vi "Color Pulse.vi"(4 "Color 2":u32(colorbox)=16711680, 5 "Style":enum16{"Sine", "Square", "Sawtooth", "Triangle"}(ring), 6 "Color 1":u32(colorbox)=16738922, 7 "Array":refnum<vi>[](array[refnum]), 10 "Pulse Period":dbl, 11 "Elapsed Time (s)":dbl) -> (2 "Color Out":u32(colorbox))   [LabVIEW 2013]
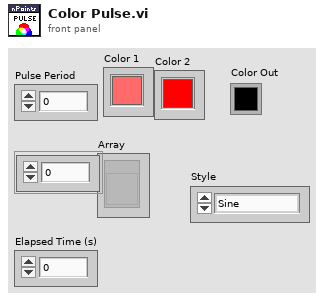
[diagram p1: front panel]
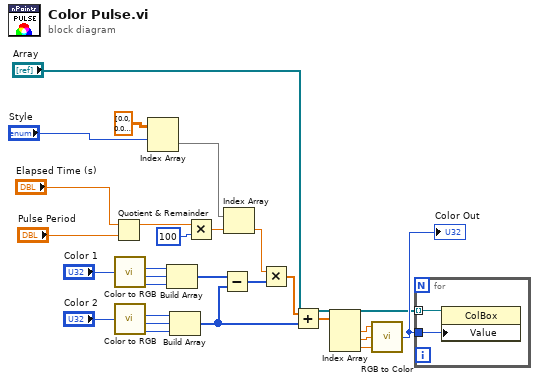
[diagram p0: block diagram]
diagram:
  n1 = Quotient & Remainder(x="Elapsed Time (s)", y="Pulse Period") -> (x-y*floor(x/y)=w23:dbl)  [unwired: 1 out]
  n2 = call <vilib>:"Color to RGB.vi"("Color"="Color 1") -> ("R"=w11:u8, "G"=w12:u8, "B"=w13:u8)  [unwired: 1 out]
  n3 = call <vilib>:"Color to RGB.vi"("Color"="Color 2") -> ("R"=w8:u8, "G"=w9:u8, "B"=w10:u8)  [unwired: 1 out]
  n4 = Index Array(array=dbl[][] [[0.0, 0.0009866357858642205, 0.0039426493427611176, 0.00885637463565564, 0.015708419435684462, 0.02447174185242318, 0.035111757055874326, 0.04758647376699021, 0.061846659978068264, 0.07783603724899246, 0.09549150281252633, 0.11474337861210537, 0.13551568628929428, 0.15772644703565564, 0.18128800512565518, 0.20610737385376343, 0.23208660251050173, 0.2591231629491424, 0.2871103542174637, 0.31593772365766104, 0.34549150281252633, 0.3756550564175726, 0.4063093427071377, 0.43733338321784787, 0.4686047402353434, 0.5, 0.5313952597646567, 0.5626666167821521, 0.5936906572928624, 0.6243449435824274, 0.6545084971874737, 0.684062276342339, 0.7128896457825363, 0.7408768370508576, 0.7679133974894983, 0.7938926261462366, 0.8187119948743449, 0.8422735529643444, 0.8644843137107058, 0.8852566213878946, 0.9045084971874737, 0.9221639627510075, 0.9381533400219317, 0.9524135262330098, 0.9648882429441257, 0.9755282581475768, 0.9842915805643155, 0.9911436253643444, 0.9960573506572389, 0.9990133642141358, 1.0, 0.9990133642141358, 0.9960573506572389, 0.9911436253643444, 0.9842915805643155, 0.9755282581475768, 0.9648882429441257, 0.9524135262330098, 0.9381533400219317, 0.9221639627510076, 0.9045084971874737, 0.8852566213878947, 0.8644843137107058, 0.8422735529643444, 0.8187119948743449, 0.7938926261462367, 0.7679133974894983, 0.7408768370508577, 0.7128896457825363, 0.6840622763423391, 0.6545084971874737, 0.6243449435824274, 0.5936906572928624, 0.5626666167821521, 0.5313952597646567, 0.5000000000000001, 0.4686047402353434, 0.4373333832178479, 0.40630934270713776, 0.3756550564175727, 0.3454915028125264, 0.3159377236576611, 0.2871103542174638, 0.2591231629491424, 0.23208660251050178, 0.2061073738537635, 0.18128800512565524, 0.1577264470356557, 0.13551568628929433, 0.11474337861210543, 0.09549150281252639, 0.07783603724899252, 0.06184665997806832, 0.04758647376699027, 0.03511175705587438, 0.024471741852423234, 0.015708419435684517, 0.008856374635655695, 0.003942649342761173, 0.0009866357858642205], [0.0, 0.0, 0.0, 0.0, 0.0, 0.0, 0.0, 0.0, 0.0, 0.0, 0.0, 0.0, 0.0, 0.0, 0.0, 0.0, 0.0, 0.0, 0.0, 0.0, 0.0, 0.0, 0.0, 0.0, 0.0, 0.0, 0.0, 0.0, 0.0, 0.0, 0.0, 0.0, 0.0, 0.0, 0.0, 0.0, 0.0, 0.0, 0.0, 0.0, 0.0, 0.0, 0.0, 0.0, 0.0, 0.0, 0.0, 0.0, 0.0, 0.0, 1.0, 1.0, 1.0, 1.0, 1.0, 1.0, 1.0, 1.0, 1.0, 1.0, 1.0, 1.0, 1.0, 1.0, 1.0, 1.0, 1.0, 1.0, 1.0, 1.0, 1.0, 1.0, 1.0, 1.0, 1.0, 1.0, 1.0, 1.0, 1.0, 1.0, 1.0, 1.0, 1.0, 1.0, 1.0, 1.0, 1.0, 1.0, 1.0, 1.0, 1.0, 1.0, 1.0, 1.0, 1.0, 1.0, 1.0, 1.0, 1.0, 1.0], [0.0, 0.010000000000000009, 0.019999999999999962, 0.030000000000000027, 0.040000000000000036, 0.050000000000000044, 0.06, 0.07, 0.08000000000000007, 0.09000000000000002, 0.10000000000000003, 0.10999999999999999, 0.12, 0.13000000000000006, 0.14, 0.15000000000000002, 0.16000000000000003, 0.16999999999999998, 0.18000000000000005, 0.19000000000000006, 0.2, 0.21000000000000002, 0.21999999999999997, 0.23000000000000004, 0.24, 0.25, 0.2600000000000001, 0.27, 0.28, 0.29, 0.30000000000000004, 0.31000000000000005, 0.32, 0.33000000000000007, 0.33999999999999997, 0.35000000000000003, 0.3600000000000001, 0.37, 0.38000000000000006, 0.38999999999999996, 0.4, 0.4100000000000001, 0.42, 0.43000000000000005, 0.43999999999999995, 0.45000000000000007, 0.4600000000000001, 0.47000000000000003, 0.4800000000000001, 0.49, 0.5, 0.51, 0.52, 0.53, 0.5399999999999999, 0.55, 0.56, 0.57, 0.5800000000000001, 0.59, 0.6, 0.6100000000000001, 0.62, 0.63, 0.6399999999999999, 0.65, 0.66, 0.6699999999999999, 0.68, 0.69, 0.7, 0.7100000000000001, 0.72, 0.73, 0.74, 0.75, 0.76, 0.77, 0.78, 0.79, 0.8, 0.81, 0.8200000000000001, 0.8300000000000001, 0.8400000000000001, 0.8500000000000001, 0.8600000000000001, 0.87, 0.8800000000000001, 0.8900000000000001, 0.9, 0.9100000000000001, 0.9199999999999999, 0.9299999999999999, 0.94, 0.95, 0.9600000000000001, 0.9700000000000002, 0.9799999999999999, 0.99], [0.0, 0.020000000000000018, 0.04000000000000009, 0.06000000000000005, 0.08000000000000007, 0.10000000000000009, 0.12000000000000005, 0.14000000000000007, 0.16000000000000003, 0.18000000000000005, 0.20000000000000007, 0.22000000000000008, 0.2400000000000001, 0.2600000000000001, 0.28, 0.30000000000000004, 0.32000000000000006, 0.3400000000000001, 0.3600000000000001, 0.3800000000000001, 0.4000000000000001, 0.4200000000000001, 0.44000000000000006, 0.4600000000000001, 0.4800000000000001, 0.5, 0.52, 0.54, 0.56, 0.5800000000000001, 0.6, 0.62, 0.64, 0.66, 0.68, 0.7, 0.72, 0.74, 0.76, 0.78, 0.8, 0.8200000000000001, 0.8400000000000001, 0.86, 0.8800000000000001, 0.9, 0.92, 0.9400000000000001, 0.96, 0.98, 1.0, 0.98, 0.96, 0.94, 0.9199999999999999, 0.8999999999999999, 0.8799999999999999, 0.86, 0.8399999999999999, 0.82, 0.8, 0.78, 0.7599999999999999, 0.7399999999999999, 0.72, 0.7, 0.6799999999999999, 0.6599999999999999, 0.6399999999999999, 0.6199999999999999, 0.6, 0.58, 0.5599999999999998, 0.5399999999999999, 0.5199999999999999, 0.49999999999999994, 0.48, 0.45999999999999985, 0.4399999999999999, 0.41999999999999993, 0.39999999999999997, 0.38, 0.3599999999999999, 0.33999999999999986, 0.31999999999999995, 0.29999999999999993, 0.27999999999999997, 0.2599999999999999, 0.23999999999999988, 0.21999999999999992, 0.19999999999999996, 0.18, 0.15999999999999986, 0.1399999999999999, 0.11999999999999994, 0.09999999999999992, 0.07999999999999996, 0.06, 0.03999999999999987, 0.01999999999999974]] ("Waveform Shapes"), index (row)="Style") -> (element=w1:dbl[])  [unwired: 1 in]
  n5 = Build Array(w11, w12, w13) -> (w14:u8[])
  n6 = Build Array(w8, w9, w10) -> (w20:u8[])
  n7 = Multiply(x=w23, y=100) -> (x*y=w4:dbl)
  n8 = Subtract(x=w14, y=w20) -> (x-y=w19:u8[])
  n9 = Index Array(array=w1, index=w4) -> (element=w24:dbl)
  n10 = Multiply(x=w24, y=w19) -> (x*y=w7:dbl[])
  n11 = Add(x=w7, y=w20) -> (x+y=w15:dbl[])
  n12 = Index Array(array=w15) -> (element #1=w16:dbl, element #2=w17:dbl, element #3=w18:dbl)  [unwired: 3 in]
  n13 = call <vilib>:"RGB to Color.vi"("B"=w18, "G"=w17, "R"=w16) -> ("Color"=w27:u32)
  "Color Out" <- w27
  n14 = for {
    tunnel: "Array" -> [w29] mode=indexing
    tunnel: w27 -> [w28]
    n15 = property class="ColBox"(reference=w29, "Value"=w28) -> ()  [unwired: 1 in, 2 out]
  }
